vi "p5_Banda_mas_interrupores.vi"() -> ()   [LabVIEW 2019]
panel:
  in  "Accion":bool=TRUE
  in  "stop":bool
  in  "Direccion":bool=TRUE
  in  "Velocidad(1m/300ms)":sgl(knob)=1.0 min=0 max=10 scale=0.0..10.0
  out "Slide":sgl(slide) scale=0.0..1200.0
  out "Tope\nDerecha":bool
  out "Tope\nIzquierda":bool
  # "Continuar"
  # "Derecha"
  # "Paro"
  # "Izquierda"
  # "Continuar"
  # "Detener"
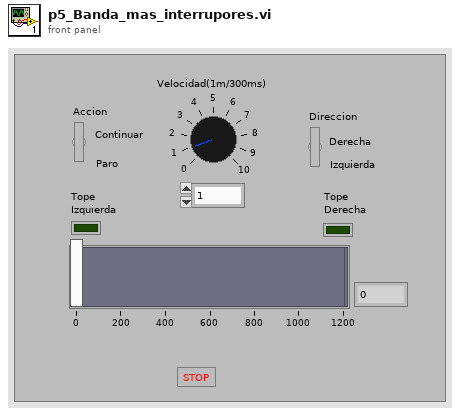
[diagram p1: front panel]
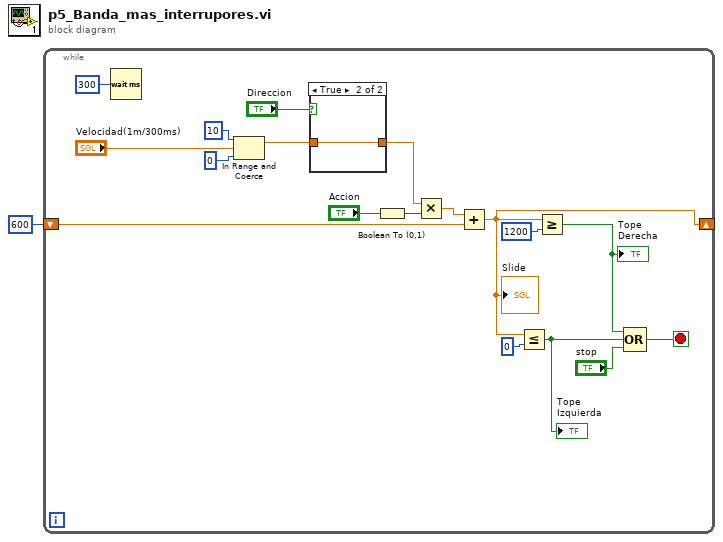
[diagram p0: block diagram]
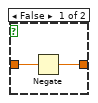
[diagram p2: hidden frame]
diagram:
  n1 = while {
    shift-right: [w7] -> _
    shift-left: i16 600 -> [w6]
    stop <- w11 stop-if-true
    n2 = Wait (ms)(milliseconds to wait=i16 300) -> ()  [unwired: 1 out]
    n3 = In Range and Coerce(upper limit=u8 10, x="Velocidad(1m/300ms)", lower limit=u8 0) -> (coerced(x)=w2:sgl)  [unwired: 1 out]
    n4 = case shown="True" "Direccion" {
      tunnel: w2 -> [w21 w22]
      tunnel: [w20 w22] -> w10
      frame False {
        n5 = Negate(x=w21) -> (-x=w20:sgl)
      }
      frame True {
      }
    }
    n6 = Boolean To (0,1)(Boolean="Accion") -> (0, 1=w9:i16)
    n7 = Multiply(x=w10, y=w9) -> (x*y=w8:sgl)
    n8 = Add(x=w8, y=w6) -> (x+y=w7:sgl)
    "Slide" <- w7
    n9 = Less Or Equal?(x=w7, y=u8 0) -> (x <= y?=w12:bool)
    "Tope\nIzquierda" <- w12
    n10 = Greater Or Equal?(x=w7, y=u16 1200) -> (x >= y?=w13:bool)
    "Tope\nDerecha" <- w13
    n11 = Compound Arithmetic op=OR(w13, w12, "stop") -> (w11:bool)
  }
